vi "GetVerticalRange.vi"(8 "error in (no error)":errorcluster, 11 "TektronixDPO_PhysicalDevice.lvclass":refnum<class "TektronixDPO_PhysicalDevice.lvclass">) -> (0 "error out":errorcluster, 3 "TektronixDPO_PhysicalDevice.lvclassOut":refnum<class "TektronixDPO_PhysicalDevice.lvclass">)   [LabVIEW 2013, in "TektronixDPO_PhysicalDevice.lvclass"]
doc: "Read from the phsyical device the offset relative to the specified channel"
uses:
  TektronixDPO_PhysicalDevice.lvclass
  TektronixDPO_PhysicalDevice.lvclass/TektronixDPO_PhysicalDevice.ctl
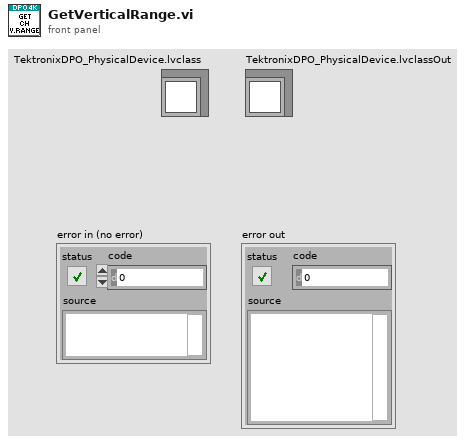
[diagram p1: front panel]
types:
  T1 = typedef "Choice80.ctl" = u16
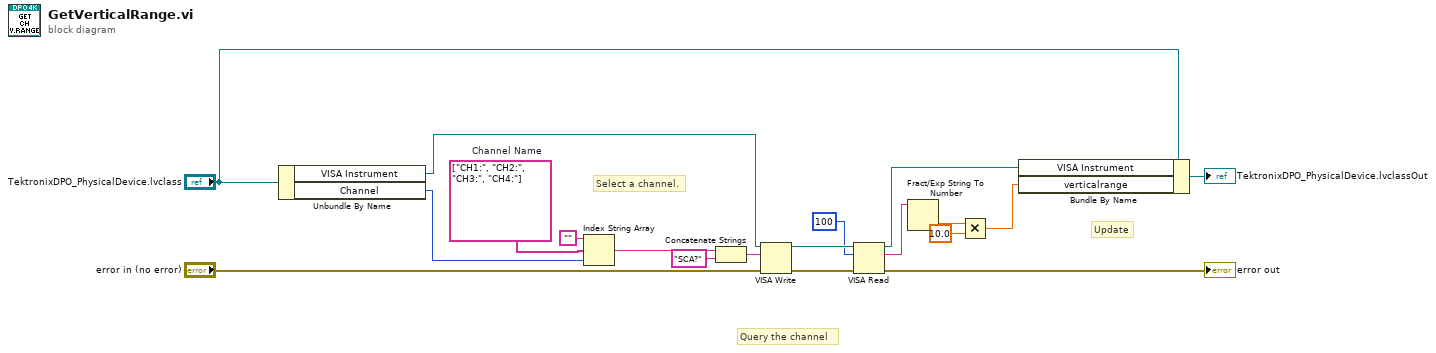
[diagram p0: block diagram]
diagram:
  w13 = string[] ["CH1:", "CH2:", "CH3:", "CH4:"]  # Channel Name
  # "Update"
  # "Query the channel"
  # "Select a channel."
  n1 = Unbundle By Name("TektronixDPO_PhysicalDevice.lvclass") -> ("VISA Instrument"=w5:refnum<visa-resource-name>, "Channel"=w7:T1)
  n2 = Index String Array(1:w7, 2:w13, 3:"") -> (0:w12:string)
  n3 = Concatenate Strings(w12, "SCA?" ("string")) -> (w10:string)
  n4 = VISA Write(VISA resource name=w5, write buffer=w10, error in (no error)="error in (no error)") -> (VISA resource name out=w17:refnum<visa-resource-name>, error out=w15:errorcluster)  [unwired: 1 out]
  n5 = VISA Read(VISA resource name=w17, byte count=u32 100, error in (no error)=w15) -> (VISA resource name out=w6:refnum<visa-resource-name>, read buffer=w2:string, error out=→"error out":errorcluster)  [unwired: 1 out]
  n6 = Fract/Exp String To Number(string=w2) -> (number=w4:dbl)  [unwired: 3 in, 1 out]
  n7 = Multiply(x=w4, y=10.0) -> (x*y=w1:dbl)
  n8 = Bundle By Name(cluster="TektronixDPO_PhysicalDevice.lvclass", "VISA Instrument"=w6, "verticalrange"=w1) -> (→"TektronixDPO_PhysicalDevice.lvclassOut":refnum<class "TektronixDPO_PhysicalDevice.lvclass">)
